vi "5-InitialAllHardware.vi"(8 "error in (no error)":errorcluster, 11 "AllControls IN":T1) -> (3 "InitalResult":bool[](array[boolean]))   [LabVIEW 2017]
uses:
  Ctrls/AllControls.ctl
  <vilib>/Instr/_visa.llb/VISA Configure Serial Port (Instr).vi
  <instrlib>/GPP/GPP.lvlib
panel:
  out "error out":errorcluster
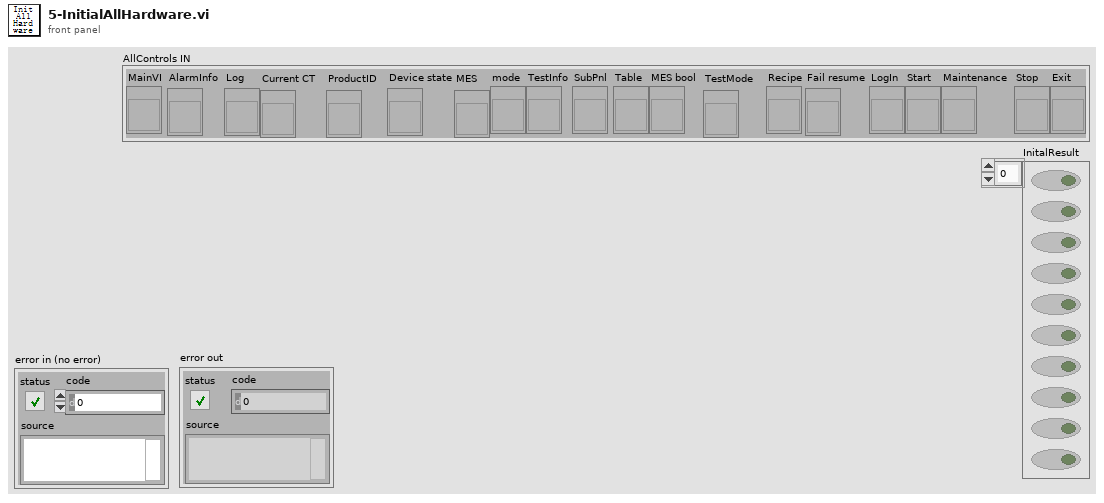
[diagram p1: front panel]
types:
  T1 = typedef "AllControls.ctl" = cluster{"MainVI":refnum<vi>, "AlarmInfo":refnum<vi>, "Log":refnum<vi>, "Current CT":refnum<vi>, "ProductID":refnum<vi>, "Device state":refnum<vi>, "MES":refnum<vi>, "mode":refnum<vi>, "TestInfo":refnum<vi>, "SubPnl":refnum<vi>, "Table":refnum<vi>, "MES bool":refnum<vi>, "TestMode":refnum<vi>, "Recipe":refnum<vi>, "Fail resume":refnum<vi>, "LogIn":refnum<vi>, "Start":refnum<vi>, "Maintenance":refnum<vi>, "Stop":refnum<vi>, "Exit":refnum<vi>}
  T2 = typedef "HD Config.ctl" = cluster{" PC":cluster{"PC Address":u8[], "PC Port":i32}, "FCO":cluster{"COM":refnum<visa-resource-name>, "Baudrate":u32}, "DC Power ":cluster{"COM":refnum<visa-resource-name>, "Baudrate":u32}, "PW3336":cluster{"COM":refnum<visa-resource-name>, "Baudrate":u32}, "Lefoo":cluster{"COM":refnum<visa-resource-name>, "Baudrate":u32}, "Tempt&Hum":cluster{"COM":refnum<visa-resource-name>, "Baudrate":u32}, "DIPC":cluster{"COM":refnum<visa-resource-name>}, "Daemon":cluster{"IP Address":string, "Port":u16, "Retry":u16}, "URAT":cluster{"COM":refnum<visa-resource-name>, "Baudrate":u32}, "Fail_resume_mode":bool, "GRR":bool}
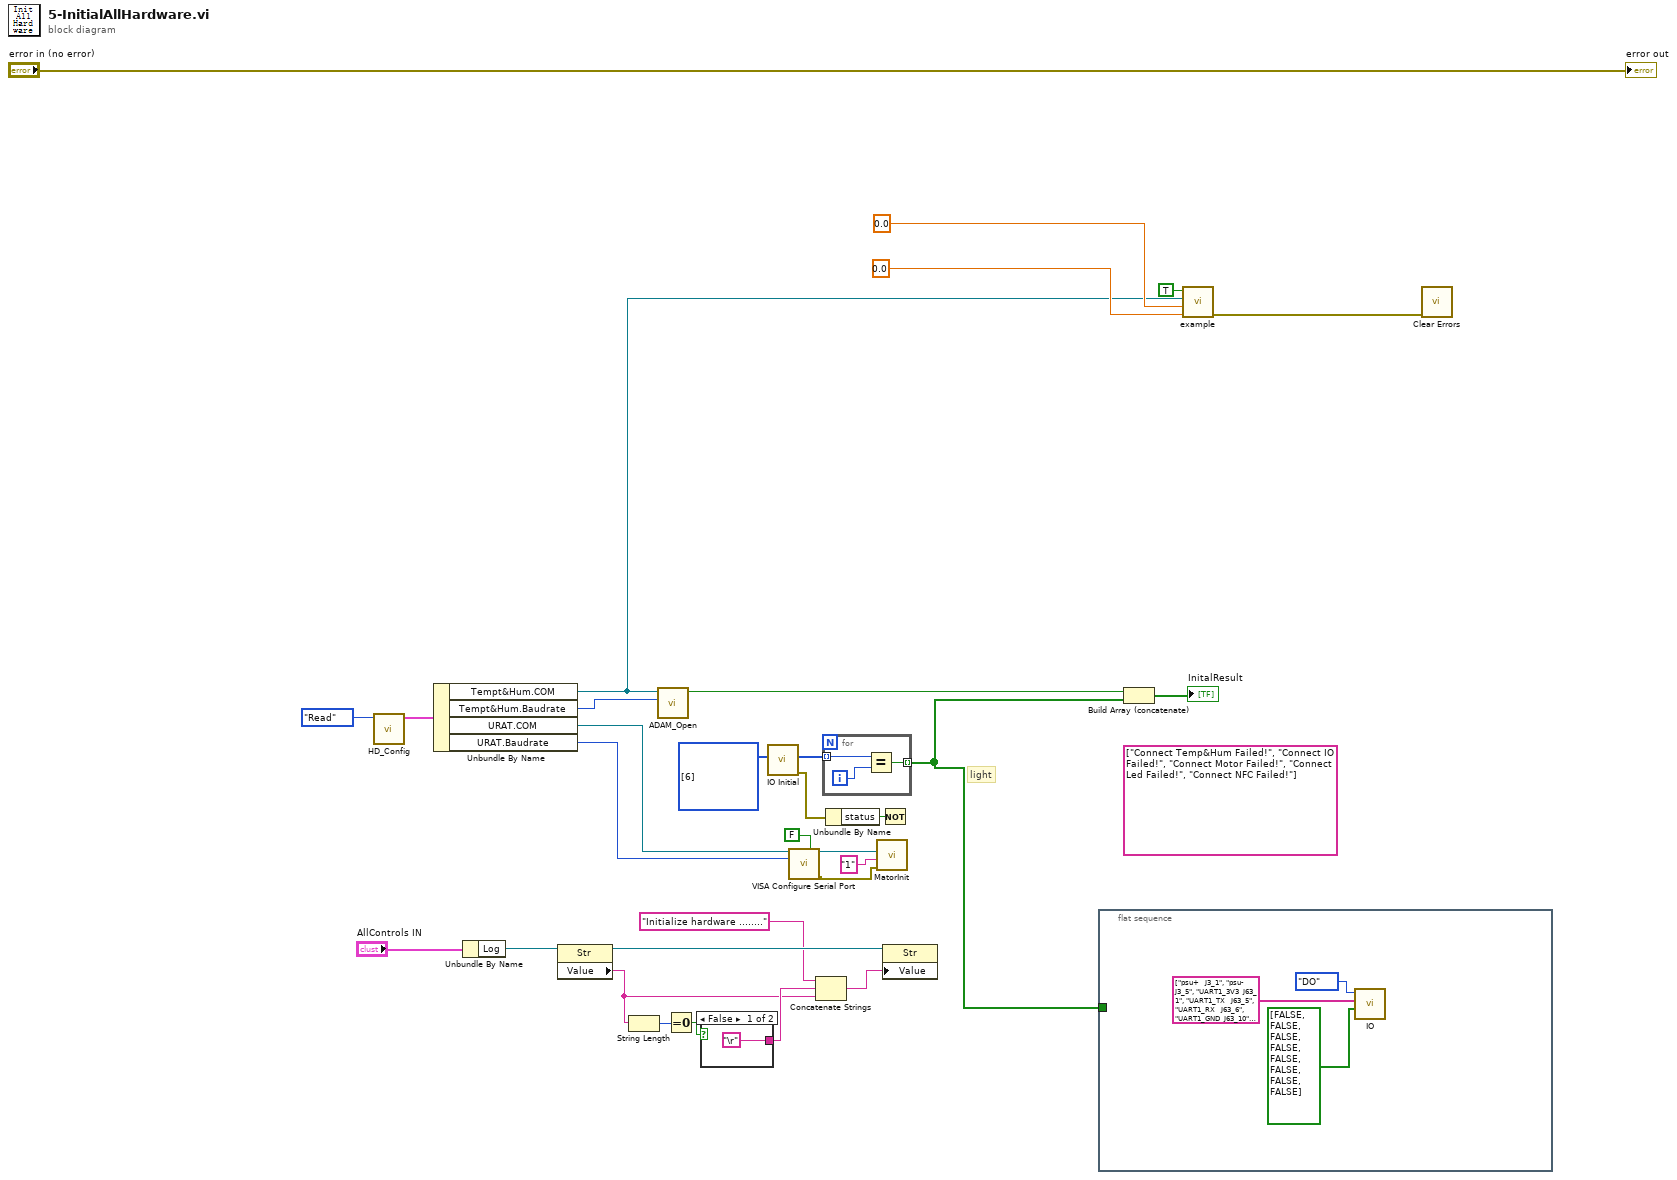
[diagram p0: block diagram]
diagram:
  (unwired) string[] ["Connect Temp&Hum Failed!", "Connect IO Failed!", "Connect Motor Failed!", "Connect Led Failed!", "Connect NFC Failed!"]
  w27 = u16[] [6] items=["PCI-7230"=6, "PCI-7432"=16, "PCI-7433"=17, "PCI-7434"=18, "PCI-7442"=37] ("CardType")
  # "light"
  n1 = call "HD_Config.vi"("Step"=enum16{"Initial", "Write", "Read"}."Read") -> ("HD Config out"=w28:T2)  [unwired: 9 in, 1 out]
  n2 = Unbundle By Name(w28) -> ("Tempt&Hum.COM"=w2:refnum<visa-resource-name>, "Tempt&Hum.Baudrate"=w14:u32, "URAT.COM"=w10:refnum<visa-resource-name>, "URAT.Baudrate"=w7:u32)
  n3 = Unbundle By Name("AllControls IN") -> ("Log"=w21:refnum<vi>)
  n4 = property class="Str"(reference=w21) -> (reference out=w23:refnum<vi>, "Value"=w16:string)  [unwired: 1 in, 1 out]
  n5 = String Length(string=w16) -> (length=w18:i32)
  n6 = call "ADAM_Open.vi"("port"=w14, "VISA resource name"=w2) -> ("status"=w13:bool)  [unwired: 8 in, 1 out]
  n7 = Equal To 0?(x=w18) -> (x = 0?=w19:bool)
  n8 = case shown="False" w19 {
    tunnel: ["\r" _] -> w17
    frame False {
    }
    frame True {
    }
  }
  n9 = call "IO Initial.vi"("CardType"=w27) -> ("error out"=w25:errorcluster, "IO f"=w26:i16[])  [unwired: 9 in]
  n10 = call-poly "VISA Configure Serial Port"("VISA resource name"=w10, "Enable Termination\nChar (T)"=FALSE ("Enable Termination\nChar (T)"), "baud rate (9600)"=w7) -> ("VISA resource name out"=w9:refnum<visa-resource-name>, "error out"=w8:errorcluster)  [unwired: 6 in, 5 out]
  n11 = Concatenate Strings("Initialize hardware ........" ("字符串"), w17, w16) -> (w20:string)
  n12 = for {
    tunnel: w26 -> [w35] mode=indexing
    tunnel: [w33] -> w6 mode=indexing
    i -> [w34]
    n13 = Equal?(x=w35, y=w34) -> (x = y?=w33:bool)
  }
  n14 = Unbundle By Name(w25) -> ("status"=w24:bool)
  n15 = call "MatorInit.vi"("错误输入（无错误）"=w8, "Chan Ident"="1", "VISA资源名称"=w9) -> ()  [unwired: 8 in, 1 out]
  n16 = Not(x=w24) -> ()  [unwired: 1 out]
  n17 = property class="Str"(reference=w23, "Value"=w20) -> ()  [unwired: 1 in, 2 out]
  n18 = flat-sequence {
    tunnel: w6 -> [_]
    frame #0 {
      n19 = call "IO.vi"("DO DATA"=bool[] [FALSE, FALSE, FALSE, FALSE, FALSE, FALSE, FALSE, FALSE] ("Writel_IO"), "IO Name"=string[] ["psu+   J3_1", "psu-   J3_5", "UART1_3V3  J63_1", "UART1_TX   J63_5", "UART1_RX   J63_6", "UART1_GND  J63_10", "PSU S+ J3_1", "PSU S- J3_5"], "IO?"=enum16{"DI", "DO"}."DO") -> ()  [unwired: 7 in, 2 out]
    }
  }
  n20 = Build Array (concatenate)(w13, w6) -> (→"InitalResult":bool[])
  n21 = call <instrlib>:"example.vi"("Current Level (A)"=0.0 ("Set Current  (A)"), "Voltage Level (V)"=0.0 ("Set Voltage  (V)"), "VISA resource name"=w2, "FLAG"=TRUE) -> ("error out"=w3:errorcluster)  [unwired: 4 in, 3 out]
  n22 = call <vilib>:"Clear Errors.vi"("error in (no error)"=w3) -> ()  [unwired: 5 in, 2 out]
  "error out" <- "error in (no error)"
